vi "2D intensity data from scan columns.vi"(10 "Graph points x,y,z":T2) -> (1 "bounds":T3, 2 "Data out":T1[][](array[typedef]))   [LabVIEW 2017, in "Scan Driver.lvclass"]
uses:
  Scan Driver.lvclass
  Instruments/Utility Classes/Readable/X.ctl
  Instruments/Utility Classes/Readable/Readable.lvclass
panel:
  in  "bounds template":T3
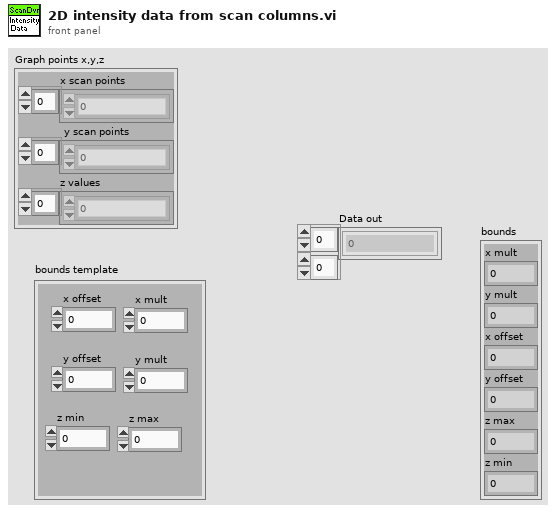
[diagram p1: front panel]
types:
  T1 = typedef "Readable.lvclass/X.ctl" = dbl
  T2 = cluster{"x scan points":T1[], "y scan points":T1[], "z values":T1[]}
  T3 = cluster{"x mult":dbl, "y mult":dbl, "x offset":dbl, "y offset":dbl, "z max":dbl, "z min":dbl}
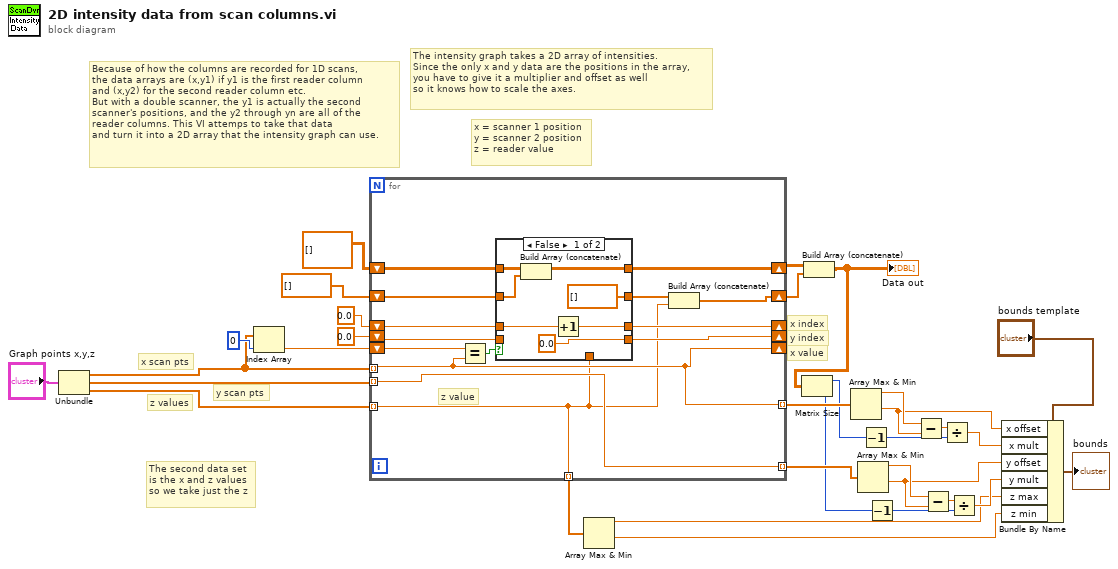
[diagram p0: block diagram]
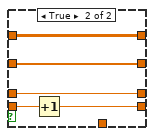
[diagram p2: hidden frame]
diagram:
  # "y scan pts"
  # "x scan pts"
  # "z values"
  # "x = scanner 1 position\ny = scanner 2 position\nz = reader value"
  # "x value"
  # "y index"
  # "x index"
  # "The second data set\nis the x and z values\nso we take just the z"
  # "Because of how the columns are recorded for 1D scans, \nthe data arrays are (x,y1) if y1 is the first reader column \nand (x,y2) for the second reader column etc. \nBut with a double scanner, the y1 is actually the second \nscanner's positions, and the y2 through yn are all of the\nreader columns. This VI attemps to take that data\nand turn it into a 2D array that the intensity graph can use."
  # "The intensity graph takes a 2D array of intensities. \nSince the only x and y data are the positions in the array, \nyou have to give it a multiplier and offset as well \nso it knows how to scale the axes."
  n1 = Unbundle("Graph points x,y,z") -> ("x scan points"=w3:T1[], "y scan points"=w2:T1[], "z values"=w1:T1[])
  n2 = Index Array(array=w3, index=0) -> (element=w13:T1)
  n3 = for {
    shift-right: [w35] -> _
    shift-left: w13 -> [w45]
    shift-right: [w36] -> _
    shift-left: 0.0 -> [w44]
    shift-right: [w39] -> _
    shift-left: 0.0 -> [w43]
    shift-right: [w40] -> w17
    shift-left: T1[][] [] ("Data out") -> [w41]
    tunnel: [w33] -> w30 mode=indexing
    shift-right: [w37] -> w16
    shift-left: dbl[] [] ("array") -> [w42]
    tunnel: [w35] -> w26 mode=indexing
    tunnel: [w34] -> w20 mode=indexing
    tunnel: w3 -> [w35] mode=indexing
    tunnel: w2 -> [w34] mode=indexing
    tunnel: w1 -> [w33] mode=indexing
    # "z value"
    n4 = Equal?(x=w45, y=w35) -> (x = y?=w46:bool)
    n5 = case shown="False" w46 {
      tunnel: [w53 w58] -> w36
      tunnel: w44 -> [w49 w58]
      tunnel: [0.0 w57] -> w39
      tunnel: w43 -> [_ w56]
      tunnel: w33 -> [_ _]
      tunnel: w42 -> [w47 w55]
      tunnel: w41 -> [w50 w54]
      tunnel: [w48 w54] -> w40
      tunnel: [dbl[] [] ("array") w55] -> w38
      frame False {
        n6 = Build Array (concatenate)(w50, w47) -> (w48:T1[][])
        n7 = Increment(x=w49) -> (x+1=w53:dbl)
      }
      frame True {
        n8 = Increment(x=w56) -> (x+1=w57:dbl)
      }
    }
    n9 = Build Array (concatenate)(w38, w33) -> (w37:T1[])
  }
  n10 = Array Max & Min(array=w30) -> (max value=w6:T1, min value=w7:T1)  [unwired: 2 out]
  n11 = Build Array (concatenate)(w17, w16) -> (w15:T1[][])
  "Data out" <- w15
  n12 = Matrix Size(0:w15) -> (1:w19:i32, 2:w18:i32)
  n13 = Array Max & Min(array=w26) -> (max value=w27:T1, min value=w10:T1)  [unwired: 2 out]
  n14 = Array Max & Min(array=w20) -> (max value=w23:T1, min value=w11:T1)  [unwired: 2 out]
  n15 = Decrement(x=w19) -> (x-1=w24:i32)
  n16 = Decrement(x=w18) -> (x-1=w21:i32)
  n17 = Subtract(x=w27, y=w10) -> (x-y=w25:T1)
  n18 = Subtract(x=w23, y=w11) -> (x-y=w22:T1)
  n19 = Divide(x=w25, y=w24) -> (x/y=w9:T1)
  n20 = Divide(x=w22, y=w21) -> (x/y=w12:T1)
  n21 = Bundle By Name(cluster="bounds template", "x offset"=w10, "x mult"=w9, "y offset"=w11, "y mult"=w12, "z max"=w6, "z min"=w7) -> (→"bounds":T3)
